vi "Handle setIDN.vi"(8 "error in (no error)":errorcluster, 10 "IDN":variant, 11 "Instrument in":refnum<class "Instrument.lvclass">) -> (0 "error out":errorcluster, 3 "Instrument out":refnum<class "Instrument.lvclass">)   [LabVIEW 2019, in "Instrument.lvlib" / "Instrument.lvclass"]
doc: "Handles setIDN command"
uses:
  Instrument.lvclass
  Typedefs/Instrument.IDN--cluster.ctl
  Instrument.lvclass/Instrument.ctl
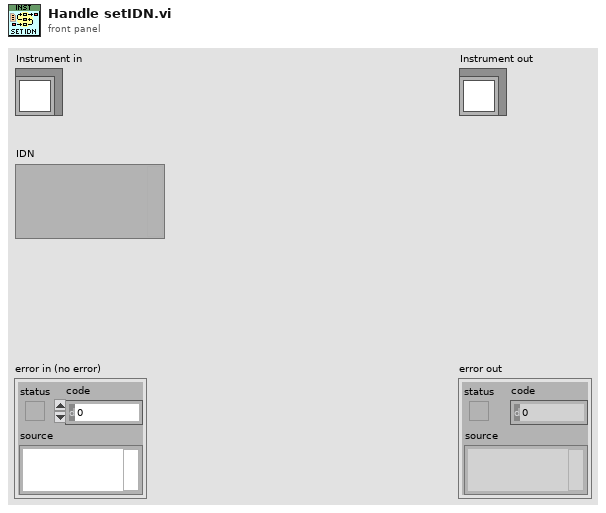
[diagram p1: front panel]
types:
  T1 = typedef "Instrument.lvlib/Instrument.lvclass/Instrument.IDN--cluster.ctl" = cluster{"vendor":string, "model":string, "serial":string, "firmware":string}
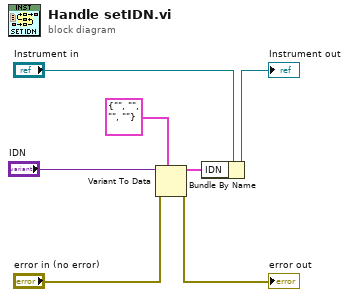
[diagram p0: block diagram]
diagram:
  n1 = Variant To Data(error in="error in (no error)", type=T1 {"vendor"="", "model"="", "serial"="", "firmware"=""} ("IDN"), Variant="IDN") -> (data=w1:T1, error out=→"error out":errorcluster)
  n2 = Bundle By Name(cluster="Instrument in", "IDN"=w1) -> (→"Instrument out":refnum<class "Instrument.lvclass">)
